vi "AKM43Lx8_InitParam8.vi"(0 "PID Loop Period":dbl=0.001 format="%#_13g", 1 "Motor Quantity":i32=8, 3 "error in (no error)":errorcluster) -> (7 "MotorCtrl":refnum<class "MotorControl.lvclass">, 10 "error out":errorcluster)   [LabVIEW 2016, in "AKM43Lx8.lvclass"]
uses:
  AKM43Lx8.lvclass
  MotorControl/MotorControl.lvclass
panel:
  in  "All Gain Schedule":T1(array[cluster])
  in  "ShaftEncCPR":dbl=2048.0 format="%#_13g"
  in  "Linearity":dbl=1.0 format="%#_13g"
  in  "Beta":dbl=0.8 format="%#_13g"
  in  "FrictionModel":cluster{"Coeff+":dbl[], "Coeff-":dbl[]}[](array[cluster])=[{"Coeff+"=[-0.12, 0.37], "Coeff-"=[-0.12, 0.37]}, {"Coeff+"=[-0.12, 0.37], "Coeff-"=[-0.12, 0.37]}, {"Coeff+"=[-0.02, 0.37], "Coeff-"=[-0.02, 0.37]}, {"Coeff+"=[-0.02, 0.37], "Coeff-"=[-0.02, 0.37]}, {"Coeff+"=[0.0, 0.37], "Coeff-"=[0.0, 0.37]}, {"Coeff+"=[0.0, 0.37], "Coeff-"=[0.0, 0.37]}, {"Coeff+"=[0.0, 0.37], "Coeff-"=[0.0, 0.37]}, {"Coeff+"=[0.0, 0.37], "Coeff-"=[0.0, 0.37]}]
  in  "MotorConstant(F/V)":dbl=43.0
  in  "Force Rate (N/min)":cluster{"ForceRateHigh":dbl, "ForceRateLow":dbl}={"ForceRateHigh"=600000.0, "ForceRateLow"=600.0} {"ForceRateHigh" format="%#_13g"; "ForceRateLow" format="%#_13g"}
  in  "TransferRatio":dbl=1.0 format="%#_13g"
  in  "output range":cluster{"output high":dbl, "output low":dbl}={"output high"=5.0, "output low"=-0.5}
  in  "setpoint range":cluster{"setpoint high":dbl, "setpoint low":dbl}={"setpoint high"=150.0, "setpoint low"=5.0}
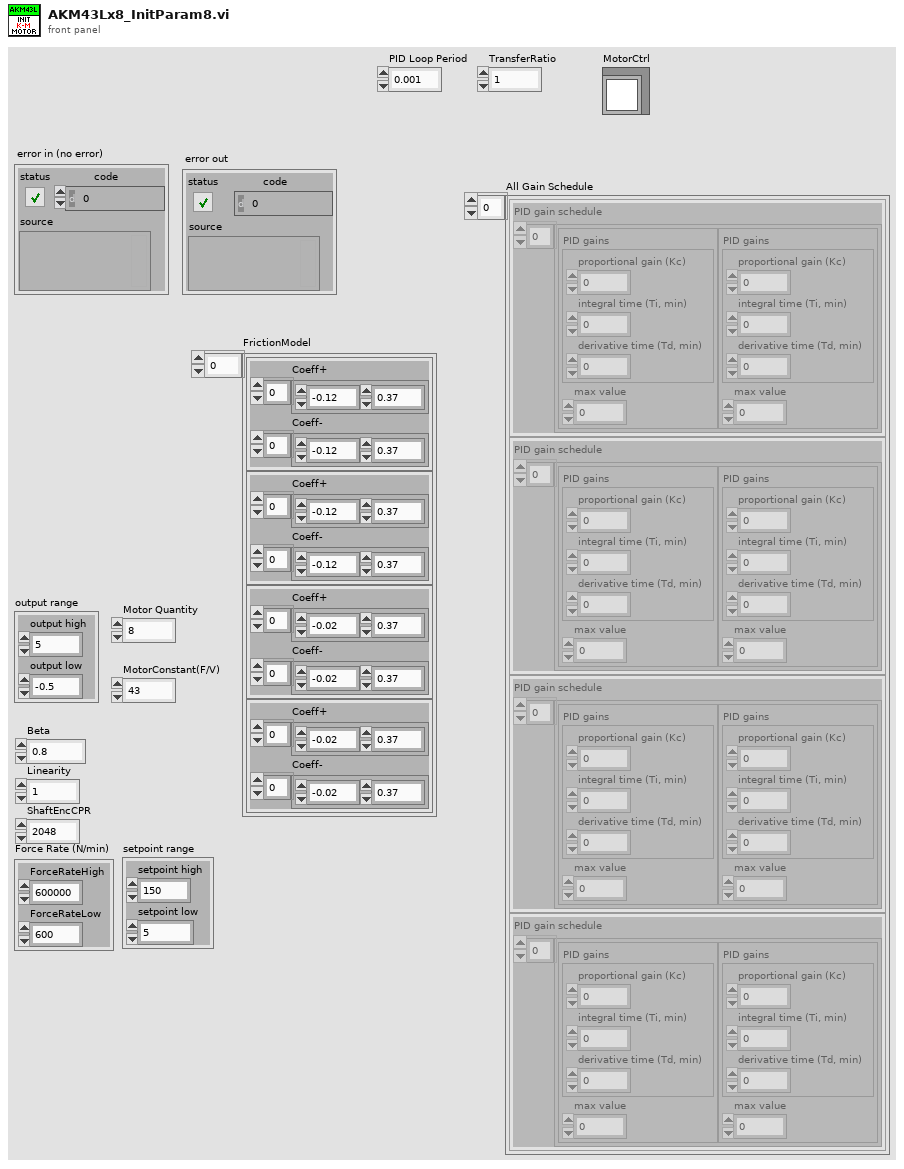
[diagram p1: front panel]
types:
  T1 = cluster{"PID gain schedule":cluster{"PID gains":cluster{"proportional gain (Kc)":dbl, "integral time (Ti, min)":dbl, "derivative time (Td, min)":dbl}, "max value":dbl}[]}[]
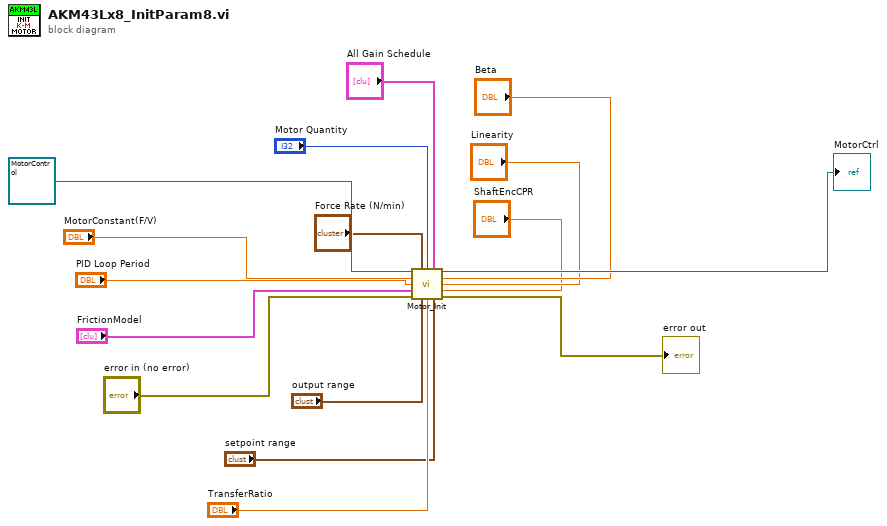
[diagram p0: block diagram]
diagram:
  n1 = call "Motor_Init.vi"("Motor Control In"=refnum<class "MotorControl.lvclass"> refnum ("MotorCtrl_In"), "Force Rate Limit (600-10000 N/min)"="Force Rate (N/min)", "Motor Quantity(1)"="Motor Quantity", "PID Params.AllGainSchedules"="All Gain Schedule", "MotorConstant(0 F/A)"="MotorConstant(F/V)", "Beta(1)"="Beta", "PID Loop Period(0.001)"="PID Loop Period", "Linearity(1)"="Linearity", "FrictionModel"="FrictionModel", "ShaftEncCPR(1000)"="ShaftEncCPR", "error in (no error)"="error in (no error)", "output range (0 - 100 N)"="output range", "TransferRatio(1)"="TransferRatio", "setpoint range (0 - 1A)"="setpoint range") -> ("Motor Control Out"=→"MotorCtrl":refnum<class "MotorControl.lvclass">, "error out"=→"error out":errorcluster)
